vi "enableMotion.vi"(8 "error in (no error)":errorcluster, 11 "Context in":refnum<class "Context.lvclass">) -> (0 "error out":errorcluster, 3 "Context out":refnum<class "Context.lvclass">)   [LabVIEW 2015]
uses:
  Model/Model/Model.lvclass
  State/State.lvclass
  Context.lvclass
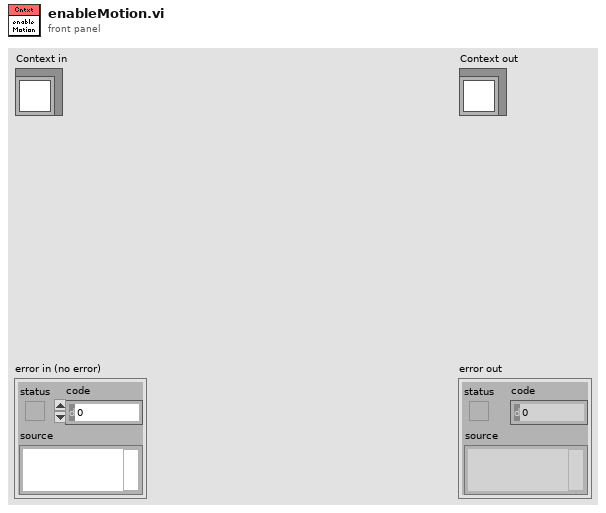
[diagram p1: front panel]
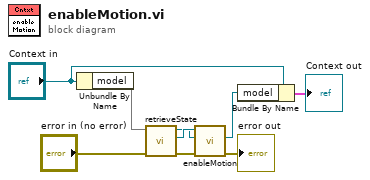
[diagram p0: block diagram]
diagram:
  n1 = Unbundle By Name("Context in") -> ("model"=w8)
  n2 = call "retrieveState.vi"("error in (no error)"="error in (no error)", "Model in"=w8) -> ("error out"=w3:errorcluster, "state"=w9:refnum<class "State.lvclass">, "Model out"=w2:refnum<class "Model.lvclass">)  [unwired: 7 in]
  n3 = call-dynamic "enableMotion.vi"("error in (no error)"=w3, "model"=w2, "State in"=w9) -> ("error out"=→"error out":errorcluster, "model 2"=w1:refnum<class "Model.lvclass">)  [unwired: 6 in, 1 out]
  n4 = Bundle By Name(cluster="Context in", "model"=w1) -> (→"Context out":cluster{})
